vi "add to repo.vi"(8 "error in":errorcluster, 9 "parent":string, 10 "serializable node":refnum<class "NISE_CEF_serializable node.lvclass">, 11 "NISE_CEF_HierarchyRepo in":refnum<class "NISE_CEF_HierarchyRepo.lvclass">) -> (0 "error out":errorcluster, 3 "NISE_CEF_HierarchyRepo out":refnum<class "NISE_CEF_HierarchyRepo.lvclass">)   [LabVIEW 2013, in "NISE_CEF_HierarchyRepo.lvclass"]
uses:
  NISE_CEF_HierarchyRepo.lvclass
  serializable node/NISE_CEF_serializable node.lvclass
  NISE_CEF_HierarchyRepo.lvclass/NISE_CEF_HierarchyRepo.ctl
  tree based serializer/NISE_CEF_TreeSerializer.lvlib
  serializable configuration/NISE_CEF_serializable configuration.lvclass
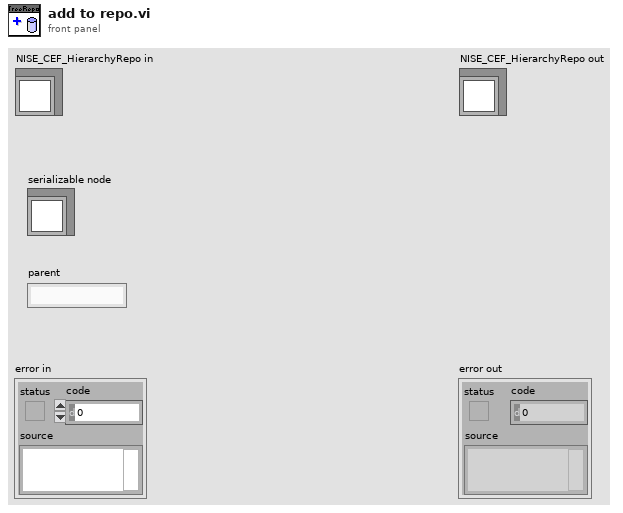
[diagram p1: front panel]
types:
  T1 = typedef "NISE_CEF_TreeSerializer.lvlib/memory hierarchy.ctl" = cluster{"root":string, "hierarchy":T2[], "instance data":refnum<class "NISE_CEF_serializable configuration.lvclass">[]}
  T2 = typedef "NISE_CEF_TreeSerializer.lvlib/hierarchy element.ctl" = cluster{"current node":string, "children":string[]}
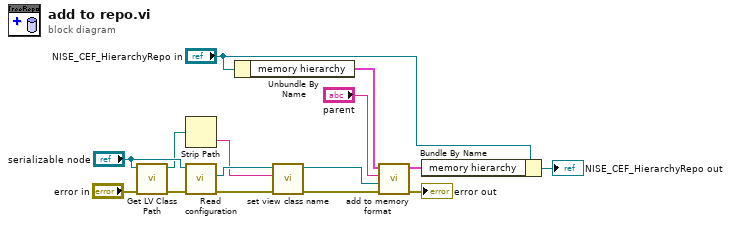
[diagram p0: block diagram]
diagram:
  n1 = call <vilib>:"Get LV Class Path.vi"("error in (no error)"="error in", "object"="serializable node") -> ("error out"=w8:errorcluster, "class path"=w6:path)  [unwired: 8 in]
  n2 = Strip Path(path=w6) -> (name=w1:string)  [unwired: 1 out]
  n3 = call-dynamic "Read configuration.vi"("error in"=w8, "NISE_CEF_serializable node in"="serializable node") -> ("error out"=w2:errorcluster, "configuration"=w3:refnum<class "NISE_CEF_serializable configuration.lvclass">)  [unwired: 7 in, 1 out]
  n4 = Unbundle By Name("NISE_CEF_HierarchyRepo in") -> ("memory hierarchy"=w12:T1)
  n5 = call "set view class name.vi"("error in"=w2, "view class"=w1, "configuration in"=w3) -> ("error out"=w5:errorcluster, "configuration out"=w4:refnum<class "NISE_CEF_serializable configuration.lvclass">)  [unwired: 7 in]
  n6 = call "add to memory format.vi"("error in"=w5, "NISE_CEF_serializable configuration in"=w4, "parent ID"="parent", "memory hierarchy in"=w12) -> ("error out"=→"error out":errorcluster, "memory hierarchy out"=w14:T1)  [unwired: 6 in]
  n7 = Bundle By Name(cluster="NISE_CEF_HierarchyRepo in", "memory hierarchy"=w14) -> (→"NISE_CEF_HierarchyRepo out":refnum<class "NISE_CEF_HierarchyRepo.lvclass">)
